vi "Interest Race_v2.vi"() -> ()   [LabVIEW 2010]
panel:
  out "Waveform Chart 2":dbl(graph)
  out "Waveform Chart":dbl(graph)
  out "Profit":dbl
  out "Profit":dbl
  in  "Daily Balance":dbl
  in  "Daily Interest Gained":dbl
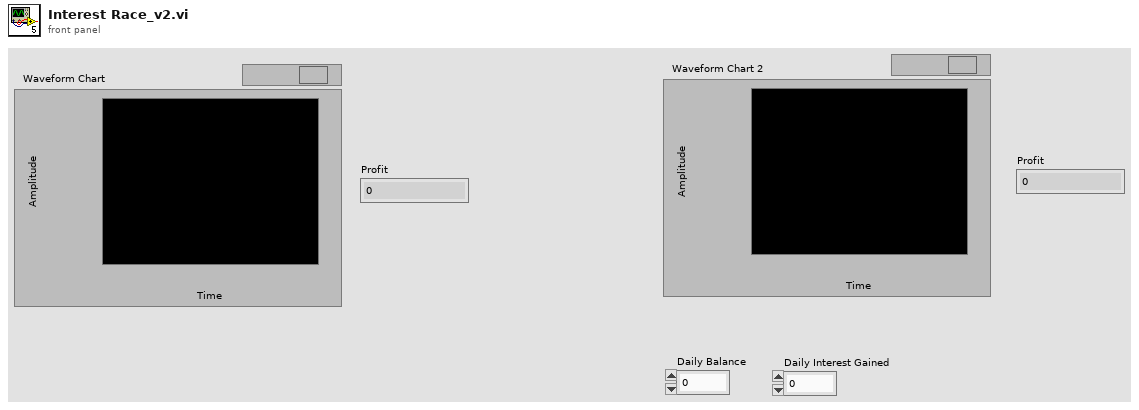
[diagram p1: front panel]
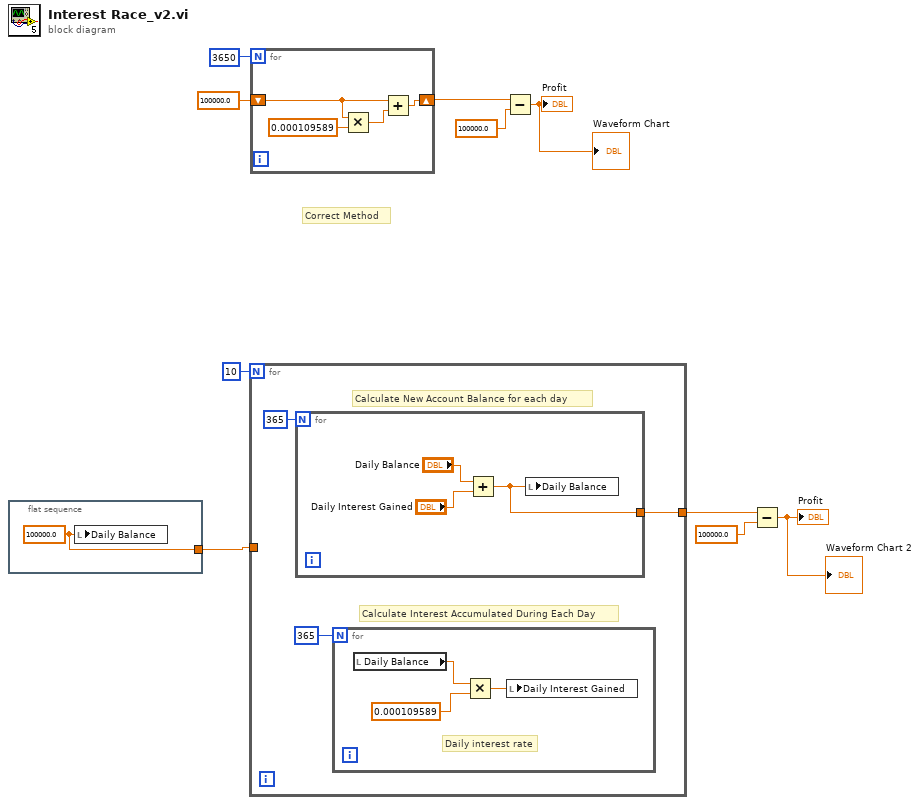
[diagram p0: block diagram]
diagram:
  # "Correct Method"
  n1 = flat-sequence {
    tunnel: [w11] -> w2
    frame #0 {
      w11 = 100000.0 ("Daily Balance")
      n2 = local write "Daily Balance"(w11) -> ()
    }
  }
  n3 = for {
    N: 10 -> [_]
    tunnel: [w12] -> w9
    tunnel: w2 -> [_]
    # "Calculate Interest Accumulated During Each Day"
    # "Calculate New Account Balance for each day"
    n4 = for {
      N: 365 -> [_]
      tunnel: [w18] -> w12
      n5 = Add(x="Daily Balance", y="Daily Interest Gained") -> (x+y=w18:dbl)
      n6 = local write "Daily Balance"(w18) -> ()
    }
    n7 = for {
      N: 365 -> [_]
      # "Daily interest rate"
      n8 = local read "Daily Balance"() -> (w17:dbl)
      n9 = Multiply(x=w17, y=0.000109589) -> (x*y=w16:dbl)
      n10 = local write "Daily Interest Gained"(w16) -> ()
    }
  }
  n11 = for {
    N: 3650 -> [_]
    shift-right: [w22] -> w5
    shift-left: 100000.0 -> [w24]
    n12 = Multiply(x=w24, y=0.000109589) -> (x*y=w23:dbl)
    n13 = Add(x=w24, y=w23) -> (x+y=w22:dbl)
  }
  n14 = Subtract(x=w5, y=100000.0) -> (x-y=→"Profit" →"Waveform Chart":dbl)
  n15 = Subtract(x=w9, y=100000.0) -> (x-y=→"Profit" →"Waveform Chart 2":dbl)
